vi "Remove Blank Space.vi"(8 "error in (no error)":errorcluster, 10 "string in":string, 11 "Setup File in":refnum<class "Setup File.lvclass">) -> (0 "error out":errorcluster, 2 "string out":string, 3 "Setup File out":refnum<class "Setup File.lvclass">)   [LabVIEW 2012, in "Setup File.lvclass"]
uses:
  Setup File.lvclass
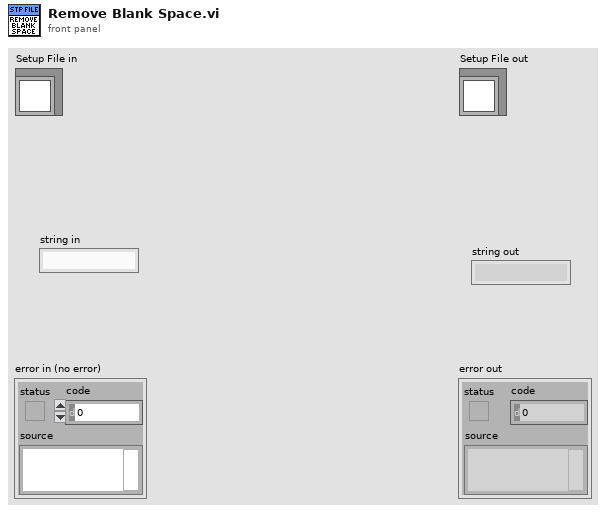
[diagram p1: front panel]
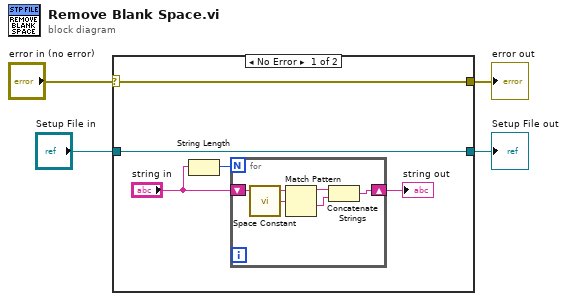
[diagram p0: block diagram]
diagram:
  n1 = case shown="No Error" "error in (no error)" {
    selector: "error in (no error)" -> [w8 w16]
    tunnel: [w8 w16] -> w2
    tunnel: [w9 w15] -> w1
    tunnel: "Setup File in" -> [w9 w15]
    frame No Error {
      n2 = String Length(string="string in") -> (length=w6:i32)
      n3 = for {
        N: w6 -> [_]
        shift-right: [w11] -> w7
        shift-left: "string in" -> [w10]
        n4 = call <vilib>:"Space Constant.vi"() -> ("String"=w12:string)
        n5 = Match Pattern(string=w10, regular expression=w12) -> (before substring=w14:string, after substring=w13:string)  [unwired: 1 in, 2 out]
        n6 = Concatenate Strings(w14, w13) -> (w11:string)
      }
      "string out" <- w7
    }
    frame Error {
    }
  }
  "error out" <- w2
  "Setup File out" <- w1
